vi "Benchmark_BuildClusterWithNames.vi"() -> ()   [LabVIEW 2020]
uses:
  _built_ppls/OpenVariant.lvlibp
panel:
  out "Cluster":variant
  out "Waveform Chart":dbl(graph)
  out "execution time per call":dbl
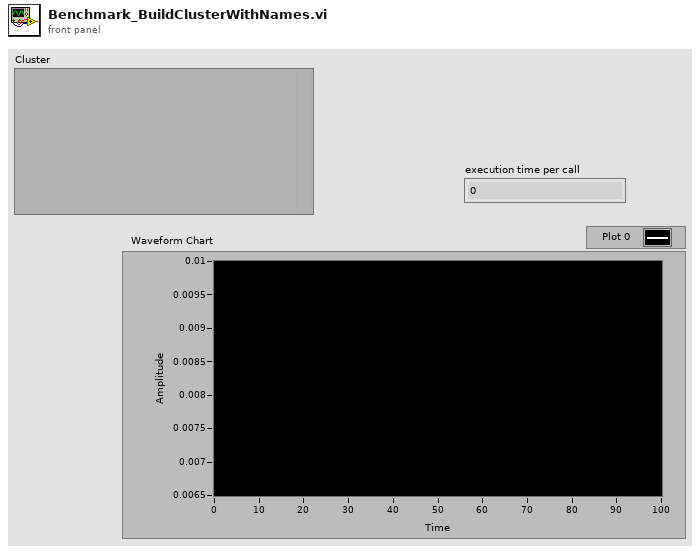
[diagram p1: front panel]
types:
  T1 = cluster{"[0]":variant, "[1]":variant, "[2]":variant, "[3]":variant, "[4]":variant, "[5]":variant, "[6]":variant, "[7]":variant, "[8]":variant, "[9]":variant, "[10]":variant, "[11]":variant, "[12]":variant, "[13]":variant, "[14]":variant, "[15]":variant, "[16]":variant, "[17]":variant, "[18]":variant, "[19]":variant, "[20]":variant, "[21]":variant, "[22]":variant, "[23]":variant, "[24]":variant, "[25]":variant, "[26]":variant, "[27]":variant, "[28]":variant, "[29]":variant, "[30]":variant, "[31]":variant, "[32]":variant, "[33]":variant, "[34]":variant, "[35]":variant, "[36]":variant, "[37]":variant, "[38]":variant, "[39]":variant, "[40]":variant, "[41]":variant, "[42]":variant, "[43]":variant, "[44]":variant, "[45]":variant, "[46]":variant, "[47]":variant, "[48]":variant, "[49]":variant, "[50]":variant, "[51]":variant, "[52]":variant, "[53]":variant, "[54]":variant, "[55]":variant, "[56]":variant, "[57]":variant, "[58]":variant, "[59]":variant, "[60]":variant, "[61]":variant, "[62]":variant, "[63]":variant, "[64]":variant, "[65]":variant, "[66]":variant, "[67]":variant, "[68]":variant, "[69]":variant, "[70]":variant, "[71]":variant, "[72]":variant, "[73]":variant, "[74]":variant, "[75]":variant, "[76]":variant, "[77]":variant, "[78]":variant, "[79]":variant, "[80]":variant, "[81]":variant, "[82]":variant, "[83]":variant, "[84]":variant, "[85]":variant, "[86]":variant, "[87]":variant, "[88]":variant, "[89]":variant, "[90]":variant, "[91]":variant, "[92]":variant, "[93]":variant, "[94]":variant, "[95]":variant, "[96]":variant, "[97]":variant, "[98]":variant, "[99]":variant, "[100]":variant, "[101]":variant, "[102]":variant, "[103]":variant, "[104]":variant, "[105]":variant, "[106]":variant, "[107]":variant, "[108]":variant, "[109]":variant, "[110]":variant, "[111]":variant, "[112]":variant, "[113]":variant, "[114]":variant, "[115]":variant, "[116]":variant, "[117]":variant, "[118]":variant, "[119]":variant, "[120]":variant, "[121]":variant, "[122]":variant, "[123]":variant, "[124]":variant, "[125]":variant, "[126]":variant, "[127]":variant, "[128]":variant, "[129]":variant, "[130]":variant, "[131]":variant, "[132]":variant, "[133]":variant, "[134]":variant, "[135]":variant, "[136]":variant, "[137]":variant, "[138]":variant, "[139]":variant, "[140]":variant, "[141]":variant, "[142]":variant, "[143]":variant, "[144]":variant, "[145]":variant, "[146]":variant, "[147]":variant, "[148]":variant, "[149]":variant, "[150]":variant, "[151]":variant, "[152]":variant, "[153]":variant, "[154]":variant, "[155]":variant, "[156]":variant, "[157]":variant, "[158]":variant, "[159]":variant, "[160]":variant, "[161]":variant, "[162]":variant, "[163]":variant, "[164]":variant, "[165]":variant, "[166]":variant, "[167]":variant, "[168]":variant, "[169]":variant, "[170]":variant, "[171]":variant, "[172]":variant, "[173]":variant, "[174]":variant, "[175]":variant, "[176]":variant, "[177]":variant, "[178]":variant, "[179]":variant, "[180]":variant, "[181]":variant, "[182]":variant, "[183]":variant, "[184]":variant, "[185]":variant, "[186]":variant, "[187]":variant, "[188]":variant, "[189]":variant, "[190]":variant, "[191]":variant, "[192]":variant, "[193]":variant, "[194]":variant, "[195]":variant, "[196]":variant, "[197]":variant, "[198]":variant, "[199]":variant, "[200]":variant, "[201]":variant, "[202]":variant, "[203]":variant, "[204]":variant, "[205]":variant, "[206]":variant, "[207]":variant, "[208]":variant, "[209]":variant, "[210]":variant, "[211]":variant, "[212]":variant, "[213]":variant, "[214]":variant, "[215]":variant, "[216]":variant, "[217]":variant, "[218]":variant, "[219]":variant, "[220]":variant, "[221]":variant, "[222]":variant, "[223]":variant, "[224]":variant, "[225]":variant, "[226]":variant, "[227]":variant, "[228]":variant, "[229]":variant, "[230]":variant, "[231]":variant, "[232]":variant, "[233]":variant, "[234]":variant, "[235]":variant, "[236]":variant, "[237]":variant, "[238]":variant, "[239]":variant, "[240]":variant, "[241]":variant, "[242]":variant, "[243]":variant, "[244]":variant, "[245]":variant, "[246]":variant, "[247]":variant, "[248]":variant, "[249]":variant, "[250]":variant, "[251]":variant, "[252]":variant, "[253]":variant, "[254]":variant, "[255]":variant}
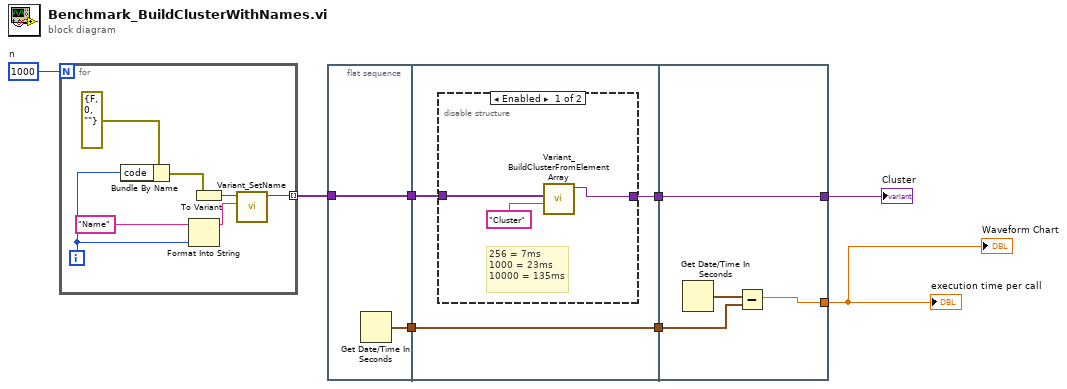
[diagram p0: block diagram]
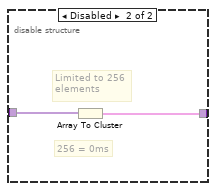
[diagram p2: hidden frame]
diagram:
  w1 = 1000  # n
  n1 = for {
    N: w1 -> [_]
    tunnel: [w12] -> w8 mode=indexing
    i -> [w10]
    n2 = Bundle By Name(cluster=errorcluster {"status"=FALSE, "code"=0, "source"=""} ("error constant"), "code"=w10) -> (w9:errorcluster)
    n3 = Format Into String(initial string="Name", w10) -> (resulting string=w13:string)  [unwired: 2 in, 1 out]
    n4 = To Variant(anything=w9) -> (Variant=w14:variant)
    n5 = call "Variant_SetName.vi"("Name"=w13, "Variant"=w14) -> ("Named Variant"=w12:variant)  [unwired: 9 in]
  }
  n6 = flat-sequence {
    tunnel: w8 -> [w17]
    tunnel: [w17] -> w7
    tunnel: [w16] -> w5
    tunnel: w7 -> [w19]
    tunnel: [w20] -> w6
    tunnel: w5 -> [w20]
    tunnel: [w18] -> w3
    tunnel: w6 -> [w28]
    tunnel: [w27] -> w4
    tunnel: w3 -> [w26]
    tunnel: [w26] -> w2
    frame #0 {
      n7 = Get Date/Time In Seconds() -> (seconds since 1Jan1904=w16:timestamp)
    }
    frame #1 {
      n8 = disable-structure shown="Enabled" {
        disable-tunnel: w19 -> [w23 w25]
        disable-tunnel: [w21 w24] -> w18
        frame Enabled {
          # "256 = 7ms\n1000 = 23ms \n10000 = 135ms"
          n9 = call "Variant_BuildClusterFromElementArray.vi"("name"="Cluster" ("initial string"), "Elements"=w23) -> ("Cluster"=w21:variant)  [unwired: 9 in]
        }
        frame Disabled {
          # "256 = 0ms"
          # "Limited to 256\nelements"
          n10 = Array To Cluster(array=w25) -> (cluster=w24:T1)
        }
      }
    }
    frame #2 {
      n11 = Get Date/Time In Seconds() -> (seconds since 1Jan1904=w29:timestamp)
      n12 = Subtract(x=w29, y=w28) -> (x-y=w27:dbl)
    }
  }
  "execution time per call" <- w4
  "Waveform Chart" <- w4
  "Cluster" <- w2
